vi "Plotter_Continuous_Receiver_Log_File.vi"(8 "error in (no error)":errorcluster, 11 "Globals":T1) -> ()   [LabVIEW 2017]
uses:
  Controls/Plotter_Globals.ctl
  Classes/ADCP.lvclass
  Controls/Plotter_Queues.ctl
  Controls/Plotter_Queue_Command_and_Data.ctl
  Controls/Plotter_Commands.ctl
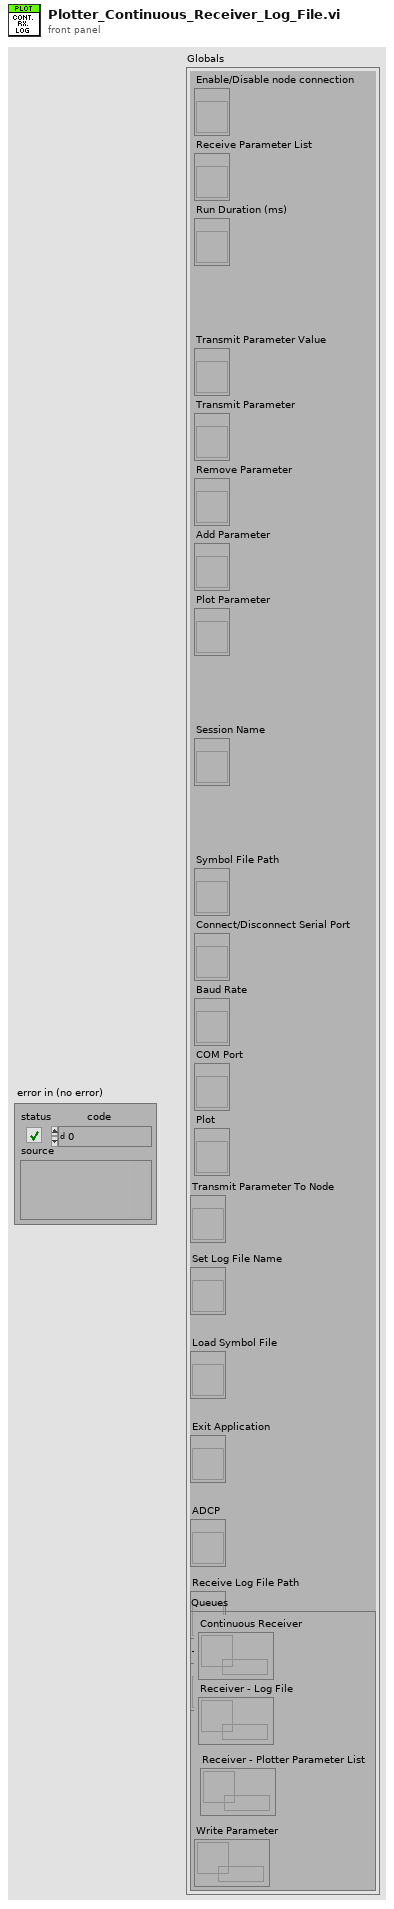
[diagram p1: front panel]
types:
  T1 = typedef "Plotter_Globals.ctl" = cluster{"Enable/Disable node connection":refnum<vi>, "Receive Parameter List":refnum<vi>, "Run Duration (ms)":refnum<vi>, "Transmit Parameter Value":refnum<vi>, "Transmit Parameter":refnum<vi>, "Remove Parameter":refnum<vi>, "Add Parameter":refnum<vi>, "Plot Parameter":refnum<vi>, "Session Name":refnum<vi>, "Symbol File Path":refnum<vi>, "Connect/Disconnect Serial Port":refnum<vi>, "Baud Rate":refnum<vi>, "COM Port":refnum<vi>, "Plot":refnum<vi>, "Transmit Parameter To Node":refnum<vi>, "Set Log File Name":refnum<vi>, "Load Symbol File":refnum<vi>, "Exit Application":refnum<vi>, "ADCP":refnum<vi>, "Transmit Log File Path":refnum<vi>, "Receive Log File Path":refnum<vi>, "Queues":T2}
  T2 = typedef "Plotter_Queues.ctl" = cluster{"Continuous Receiver":refnum<queue>, "Receiver - Log File":refnum<queue>, "Receiver - Plotter Parameter List":refnum<queue>, "Write Parameter":refnum<queue>}
  T3 = typedef "Plotter_Queue_Command_and_Data.ctl" = cluster{"Commands":T4, "Data":variant}
  T4 = typedef "Plotter_Commands.ctl" = enum16{"Idle", "Cont_RX_Open_Node", "Cont_RX_Flush_Serial_Port", "Cont_Rx_Log_Write", "Plot_Update", "Exit"}
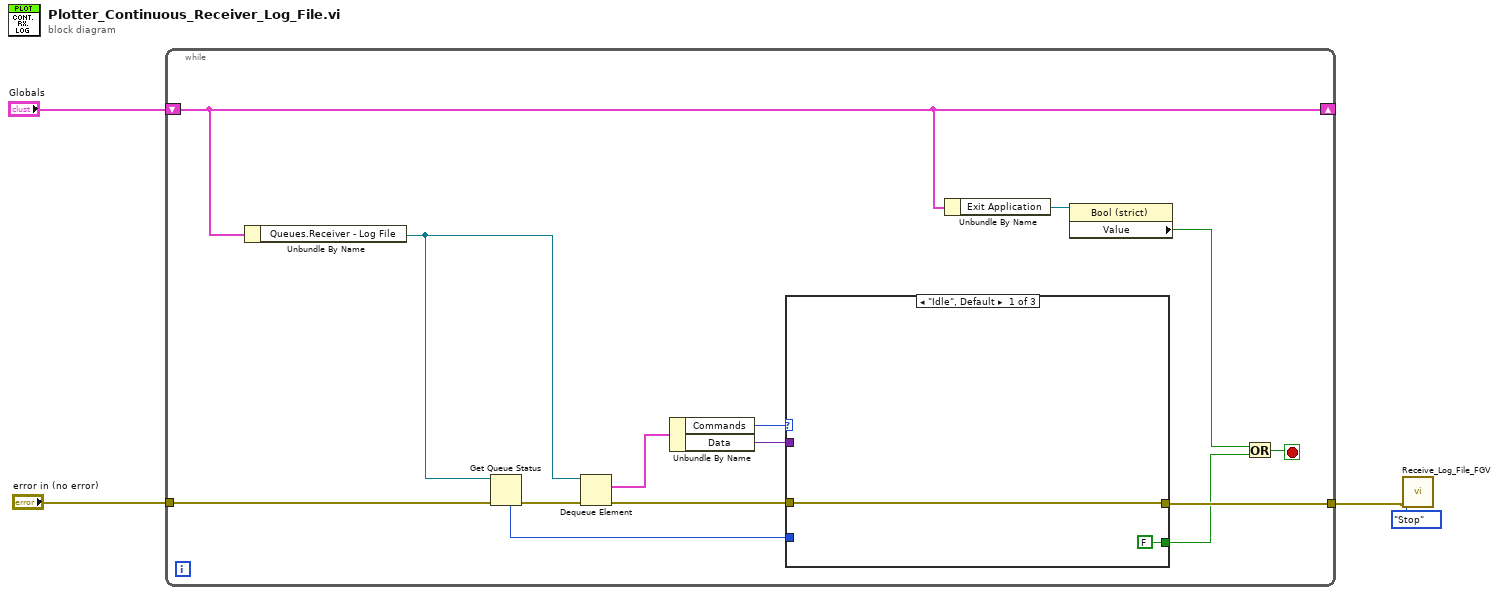
[diagram p0: block diagram]
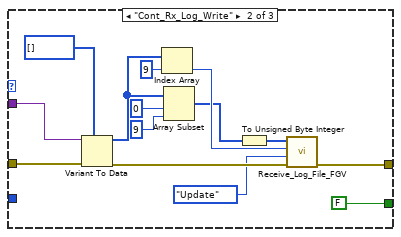
[diagram p2: hidden frame]
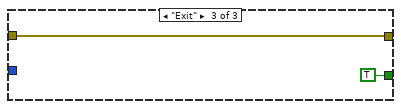
[diagram p3: hidden frame]
diagram:
  n1 = while {
    shift-right: [w7] -> _
    shift-left: "Globals" -> [w7]
    tunnel: "error in (no error)" -> [w13]
    tunnel: [w14] -> w2
    stop <- w9 stop-if-true
    n2 = Unbundle By Name(w7) -> ("Queues.Receiver - Log File"=w11:refnum<queue>)
    n3 = Get Queue Status(queue=w11, error in (no error)=w13) -> (error out=w12:errorcluster, # elements in queue=w10:i32)  [unwired: 1 in, 6 out]
    n4 = Dequeue Element(queue=w11, error in (no error)=w12) -> (element=w16:T3, error out=w18:errorcluster)  [unwired: 1 in, 2 out]
    n5 = Unbundle By Name(w16) -> ("Commands"=w17:T4, "Data"=w15:variant)
    n6 = case shown="\"Idle\", Default" w17 {
      tunnel: w18 -> [w20 w34 w36]
      tunnel: w15 -> [_ w33 _]
      tunnel: [FALSE FALSE TRUE] -> w8
      tunnel: [w20 w22 w36] -> w14
      tunnel: w10 -> [_ _ _]
      frame "Idle", Default {
      }
      frame "Cont_Rx_Log_Write" {
        n7 = Variant To Data(error in=w34, type=u32[] [], Variant=w33) -> (data=w28:u32[], error out=w31:errorcluster)
        n8 = Index Array(array=w28, index=9) -> (element=w29:u32)
        n9 = Array Subset(array=w28, index=0, length=9) -> (w25:u32[])
        n10 = To Unsigned Byte Integer(number=w25) -> (unsigned 8bit integer=w24:u8[])
        n11 = call "Receive_Log_File_FGV.vi"("error in (no error)"=w31, "Command"=enum16{"Initialize", "Update", "Stop"}."Update", "Time (ms)"=w29, "Processed bytes"=w24) -> ("error out"=w22:errorcluster)  [unwired: 6 in, 1 out]
      }
      frame "Exit" {
      }
    }
    n12 = Unbundle By Name(w7) -> ("Exit Application"=w6:refnum<vi>)
    n13 = property class="Bool (strict)"(reference=w6) -> ("Value"=w5:bool)  [unwired: 1 in, 2 out]
    n14 = Or(x=w5, y=w8) -> (x .or. y?=w9:bool)
  }
  n15 = call "Receive_Log_File_FGV.vi"("error in (no error)"=w2, "Command"=enum16{"Initialize", "Update", "Stop"}."Stop") -> ()  [unwired: 8 in, 2 out]
